vi "Write Offset and Multiplier.vi"(5 "Offset and Multiplier":cluster{"Offset":dbl, "Multiplier":dbl}, 9 "GraphScale in":refnum<class "GraphScale.lvclass">) -> (3 "GraphScale out":refnum<class "GraphScale.lvclass">)   [LabVIEW 2014, in "Raspberry Pi Compatible Compiler for LabVIEW.lvlib" / "GraphScale.lvclass"]
uses:
  GraphScale.lvclass
  GraphScale.lvclass/GraphScale.ctl
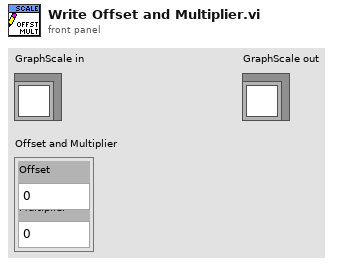
[diagram p1: front panel]
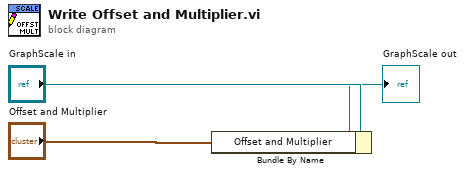
[diagram p0: block diagram]
diagram:
  n1 = Bundle By Name(cluster="GraphScale in", "Offset and Multiplier"="Offset and Multiplier") -> (→"GraphScale out":refnum<class "GraphScale.lvclass">)
